vi "Oven Temp Monitor.vi"() -> ()   [LabVIEW 2016]
doc: "Monitors temperature of Cesium oven in Source A via Omega CNi854 Monitor/Controller"
panel:
  in  "Tab Control":enum32{"Main", "Config"}(tab)
  out "Oven Temperature":dbl(graph)
  out "Oven Temp (°C)":dbl
  in  "stop":bool
  out "Omega T error":errorcluster
  in  "Omega VISA resource":refnum<visa-resource-name>="TCPIP0::192.168.1.173::2000::SOCKET"
  out "Omega read buffer":string
  out "Read errors":i32
  in  "Wait (ms)":u32=500
  in  "byte count":u32=15
  out "Omega Iteration":i32
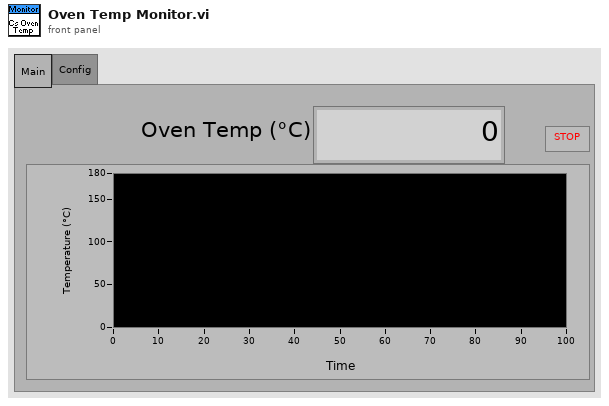
[diagram p1: front panel]
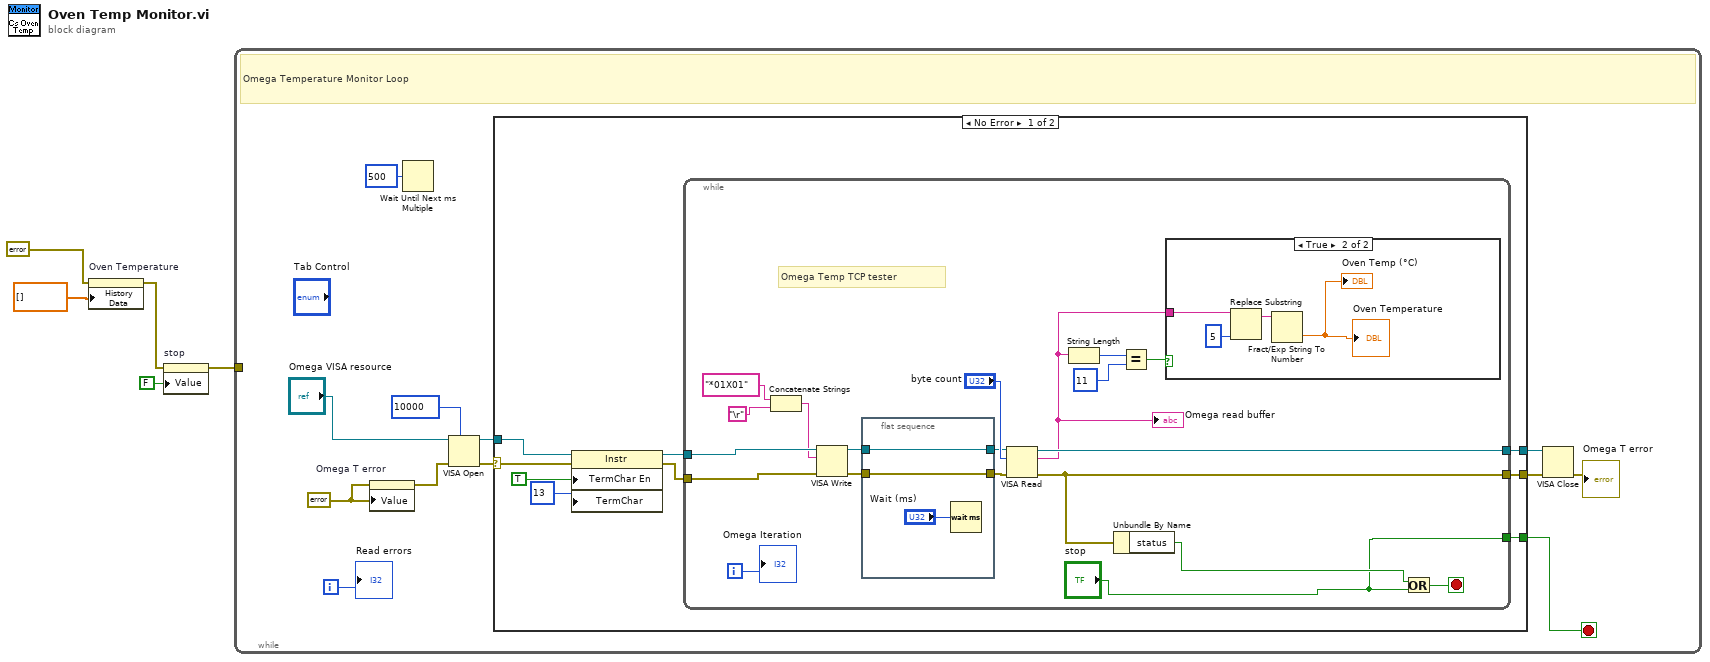
[diagram p0: block diagram]
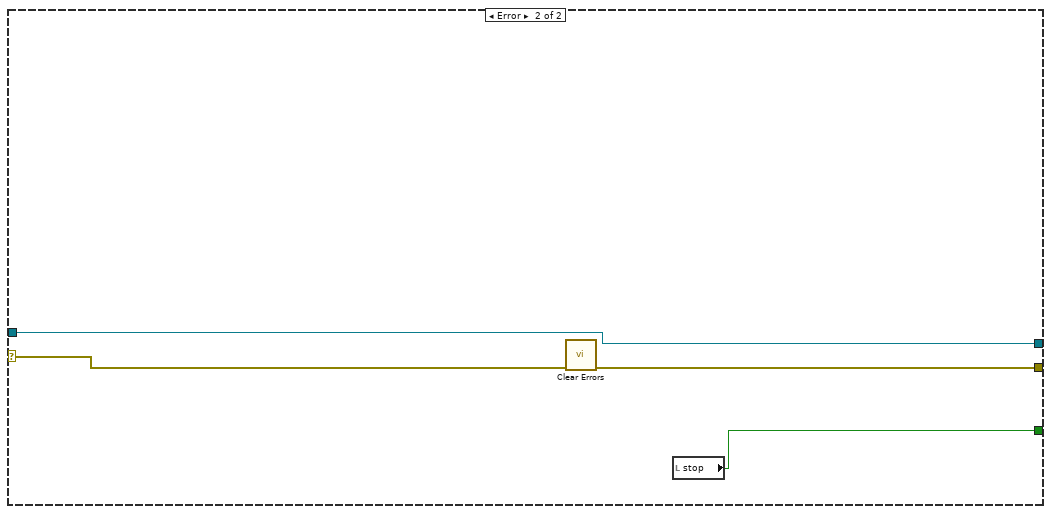
[diagram p3: hidden frame]
diagram:
  n1 = property on="Oven Temperature" class="WFChart (strict)"(error in=errorcluster {"status"=FALSE, "code"=0, "source"=""} ("error in (no error)"), "History Data"=dbl[] []) -> (error out=w3:errorcluster)  [unwired: 1 in, 1 out]
  n2 = property on="stop" class="Bool (strict)"(error in=w3, "Value"=FALSE ("stop")) -> (error out=w1:errorcluster)  [unwired: 1 in, 1 out]
  n3 = while {
    tunnel: w1 -> [_]
    i -> [w9]
    stop <- w10 stop-if-true
    w12 = errorcluster {"status"=FALSE, "code"=0, "source"=""} ("error in (no error)")
    # "Omega Temperature Monitor Loop"
    n4 = property on="Omega T error" class="Clust (strict)"(error in=w12, "Value"=w12) -> (error out=w13:errorcluster)  [unwired: 1 in, 1 out]
    n5 = Wait Until Next ms Multiple(millisecond multiple=u32 500) -> ()  [unwired: 1 out]
    n6 = VISA Open(timeout (0)=u32 10000 ("VISA Open timeout (0)"), error in (no error)=w13, VISA resource name="Omega VISA resource") -> (VISA resource name=w17:refnum<visa-resource-name>, error out=w8:errorcluster)  [unwired: 2 in]
    n7 = case shown="No Error" w8 {
      selector: w8 -> [w19 w56]
      tunnel: w17 -> [w24 w57]
      tunnel: [w26 w57] -> w16
      tunnel: [w25 w55] -> w15
      tunnel: [w20 w54] -> w10
      frame No Error {
        n8 = property class="Instr"(reference=w24, error in=w19, "TermChar En"=TRUE ("Message Based Settings:Termination Character Enable"), "TermChar"=u8 13 ("Message Based Settings:Termination Character")) -> (reference out=w23:refnum<visa-resource-name>, error out=w18:errorcluster)
        n9 = while {
          tunnel: w23 -> [w42]
          tunnel: [w46] -> w26
          tunnel: w18 -> [w37]
          tunnel: [w45] -> w25
          tunnel: ["stop"] -> w20
          i -> [w43]
          stop <- w44 stop-if-true
          # "Omega Temp TCP tester"
          n10 = Concatenate Strings("*01X01" ("data in"), "\r") -> (w39:string)
          n11 = VISA Write(VISA resource name=w42, write buffer=w39, error in (no error)=w37) -> (VISA resource name out=w30:refnum<visa-resource-name>, error out=w32:errorcluster)  [unwired: 1 out]
          n12 = flat-sequence {
            tunnel: w32 -> [w49]
            tunnel: [w49] -> w31
            tunnel: w30 -> [w48]
            tunnel: [w48] -> w29
            frame #0 {
              n13 = Wait (ms)(milliseconds to wait="Wait (ms)") -> ()  [unwired: 1 out]
            }
          }
          n14 = VISA Read(VISA resource name=w29, byte count="byte count", error in (no error)=w31) -> (VISA resource name out=w46:refnum<visa-resource-name>, read buffer=w33:string, error out=w45:errorcluster)  [unwired: 1 out]
          "Omega read buffer" <- w33
          n15 = String Length(string=w33) -> (length=w36:i32)
          n16 = Unbundle By Name(w45) -> ("status"=w28:bool)
          n17 = Equal?(x=w36, y=11) -> (x = y?=w34:bool)
          n18 = case shown="True" w34 {
            tunnel: w33 -> [_ w50]
            frame False {
            }
            frame True {
              n19 = Replace Substring(2:5 ("length (len. of substring)"), 5:w50) -> (1:w51:string)  [unwired: 2 in, 1 out]
              n20 = Fract/Exp String To Number(string=w51) -> (number=→"Oven Temp (°C)" →"Oven Temperature":dbl)  [unwired: 3 in, 1 out]
            }
          }
          n21 = Or(x=w28, y="stop") -> (x .or. y?=w44:bool)
          "Omega Iteration" <- w43
        }
      }
      frame Error {
        n22 = call <vilib>:"Clear Errors.vi"("error in (no error)"=w56) -> ("error out"=w55:errorcluster)  [unwired: 5 in, 1 out]
        n23 = local read "stop"() -> (w54:bool)
      }
    }
    n24 = VISA Close(VISA resource name=w16, error in (no error)=w15) -> (error out=→"Omega T error":errorcluster)
    "Read errors" <- w9
  }
